vi "Offline_Analysis_SVM_분석기_woF4.vi"(0 "LDA_matrix":path caption="LDA_matrix.txt", 1 "Target":path, 2 "Nontarget":path, 3 "DIscard Channel Info":i32[](array[numeric]), 5 "Target_order.txt":path, 7 "mius_flash_order":path, 9 "Brain":path, 11 "svm_model_file":string, 12 "피험자이름":string="홍길동", 13 "Save_path":string) -> ()   [LabVIEW 2014]
uses:
  <vilib>/Utility/file.llb/Read From Spreadsheet File (DBL).vi
  <vilib>/Analysis/Matrix/Numeric/Conversions/Array To Matrix - RA2.vi
  <vilib>/Analysis/Matrix/Numeric/Conversions/Array To Matrix - RA.vi
  <vilib>/Utility/file.llb/Read From Spreadsheet File (I64).vi
  <vilib>/Utility/file.llb/Write To Spreadsheet File (DBL).vi
  <vilib>/Utility/file.llb/Write To Spreadsheet File (I64).vi
  <vilib>/Utility/file.llb/Write To Spreadsheet File (string).vi
  <vilib>/Analysis/Matrix/NI_Matrix.lvlib
panel:
  out "ACC":i16
  in  "Channel selection":bool[](array[boolean])=[TRUE, TRUE, TRUE, TRUE, TRUE, TRUE, TRUE, TRUE, TRUE, TRUE, TRUE]
  out "Target_order":i64[](array[numeric])
  out "Selected_Target":i32[](array[numeric])
  out "Accuracy":i16[](array[numeric])
  out "error out":errorcluster
  in  "Random_num":i32=6
  in  "Flash_Repeat":i32=20
  in  "Frame_Length":i32=10
  in  "Sampling_Rate":dbl=250.0
  # "ERP_Parameter안씀. LDA바로 집어넣으면 됨"
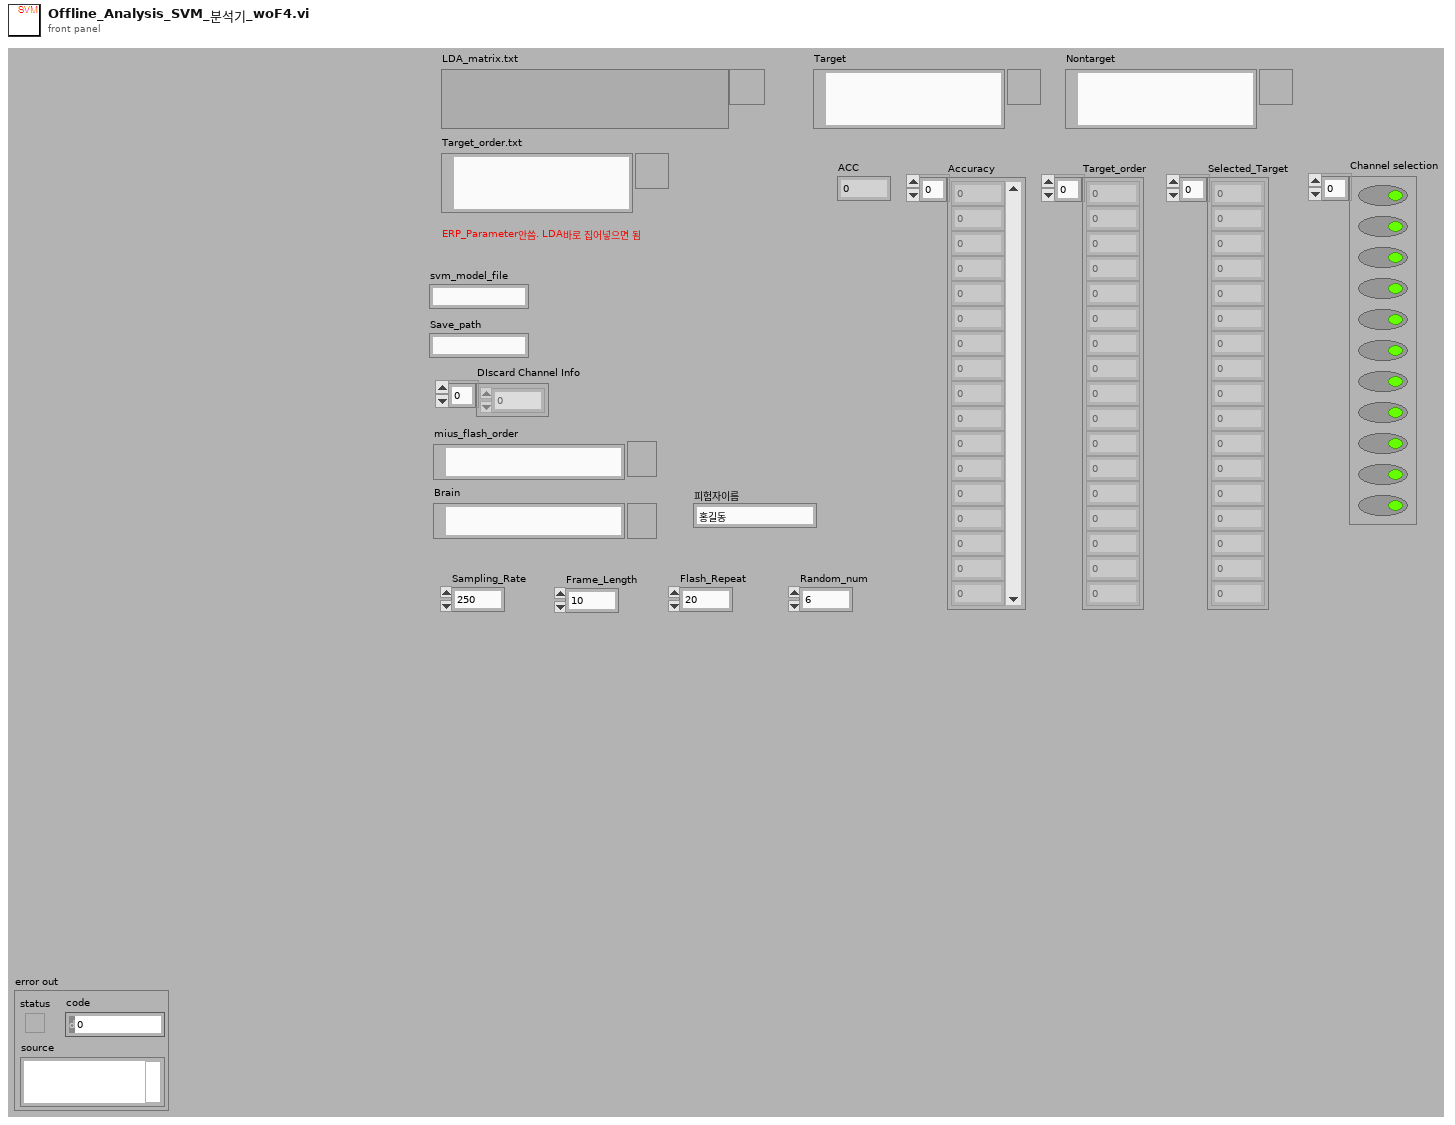
[diagram p1: front panel]
types:
  T1 = typedef "NI_Matrix.lvlib/RealMatrix.ctl" = dbl[][]
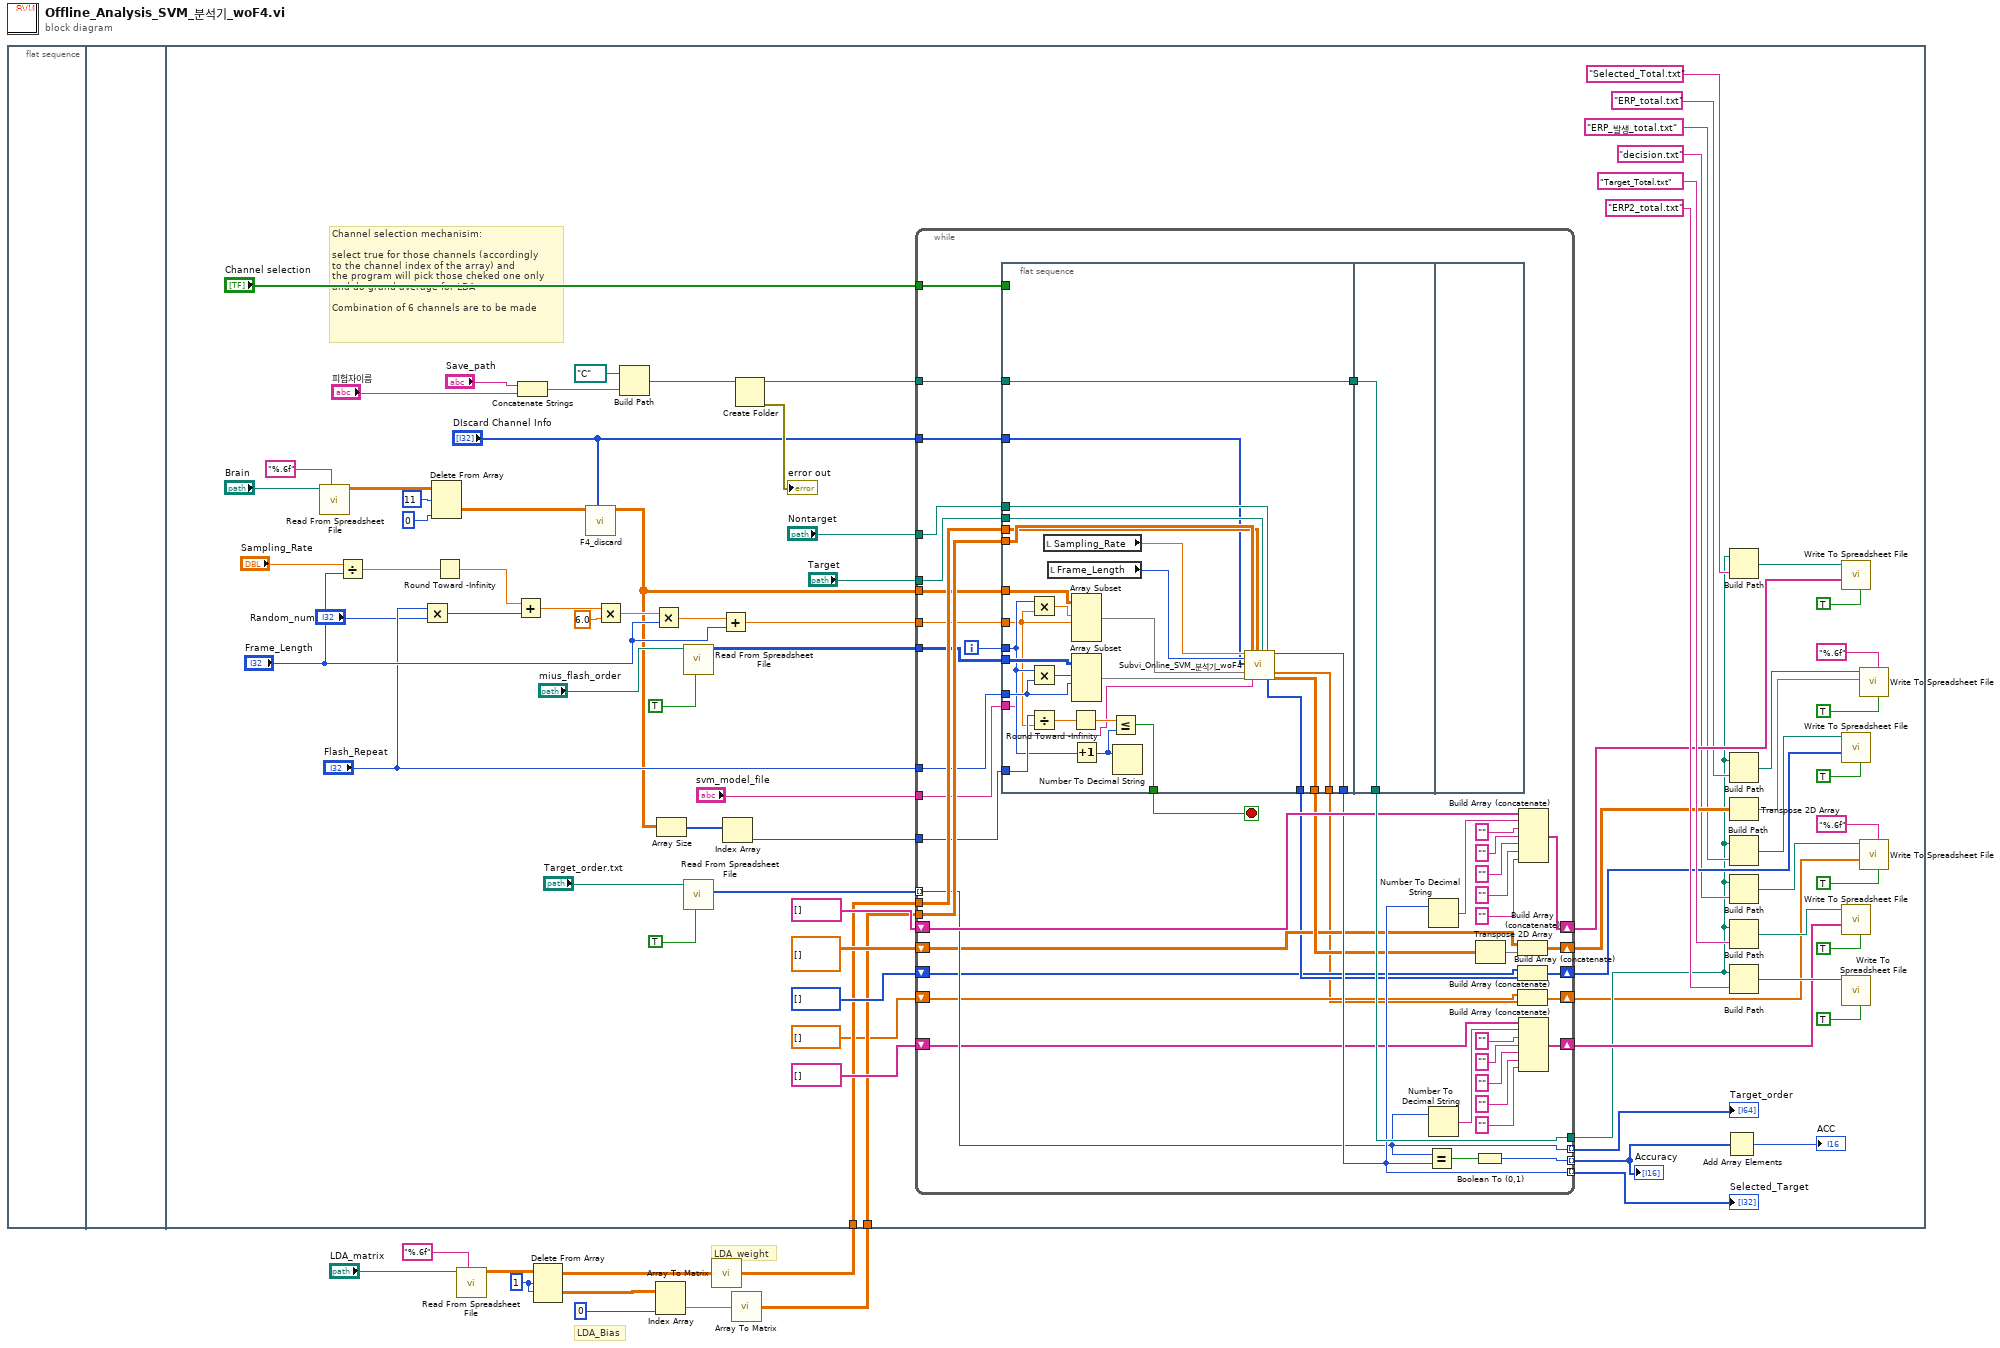
[diagram p0: block diagram]
diagram:
  w5 = 1 ("인덱스 (행)")
  # "LDA_Bias"
  # "LDA_weight"
  n1 = flat-sequence {
    tunnel: w2 -> [w27]
    tunnel: w1 -> [w26]
    frame #0 {
    }
    frame #1 {
    }
    frame #2 {
      # "Channel selection mechanisim:\n\nselect true for those channels (accordingly\nto the channel index of the array) and \nthe program will pick those cheked one only\nand do grand average for LDA\n\nCombination of 6 channels are to be made"
      n2 = call-poly <vilib>:"Read From Spreadsheet File.vi"("format (%.3f)"="%.6f", "file path (dialog if empty)"="Brain") -> ("all rows"=w65:dbl[][])  [unwired: 5 in, 4 out]
      n3 = Divide(x="Sampling_Rate", y="Frame_Length") -> (x/y=w71:dbl)
      n4 = Multiply(x="Flash_Repeat", y="Random_num") -> (x*y=w74:i32)
      n5 = Delete From Array(array=w65, length=11 ("길이"), index (col)=0 ("비활성화된 인덱스 (열)")) -> (deleted portion=w25:dbl[][])  [unwired: 1 in, 1 out]
      n6 = Round Toward -Infinity(1:w71) -> (0:w73:dbl)
      n7 = Add(x=w73, y=w74) -> (x+y=w76:dbl)
      n8 = Concatenate Strings("Save_path", "피험자이름") -> (w17:string)
      n9 = call "F4_discard.vi"("DIscard Channel Info"="DIscard Channel Info", "Array"=w25) -> ("array w/ subset deleted"=w12:dbl[][])  [unwired: 9 in]
      n10 = Multiply(x=w76, y=6.0) -> (x*y=w78:dbl)
      n11 = Build Path(base path=path "C:/" ("path"), name or relative path=w17) -> (appended path=w83:path)
      n12 = Multiply(x=w78, y="Frame_Length") -> (x*y=w80:dbl)
      n13 = Array Size(array=w12) -> (size(s)=w68:i32[])
      n14 = call-poly <vilib>:"Read From Spreadsheet File.vi"("transpose (no:F)"=TRUE, "file path (dialog if empty)"="mius_flash_order") -> ("all rows"=w67:i64[][])  [unwired: 5 in, 4 out]
      n15 = call-poly <vilib>:"Read From Spreadsheet File.vi"("transpose (no:F)"=TRUE, "file path (dialog if empty)"="Target_order.txt") -> ("first row"=w59:i64[])  [unwired: 5 in, 4 out]
      n16 = Add(x=w80, y="Frame_Length") -> (x+y=w81:dbl)
      n17 = Index Array(array=w68) -> (element=w69:i32)  [unwired: 1 in]
      n18 = Create Folder(path (use dialog)=w83) -> (created path=w85:path, error out=→"error out":errorcluster)  [unwired: 2 in, 1 out]
      n19 = while {
        tunnel: w26 -> [w134]
        tunnel: w27 -> [w133]
        tunnel: w12 -> [w131]
        tunnel: w67 -> [w130]
        tunnel: w69 -> [w132]
        tunnel: w81 -> [w128]
        tunnel: "Flash_Repeat" -> [w129]
        tunnel: w85 -> [w127]
        tunnel: w59 -> [w104] mode=indexing
        tunnel: [w124] -> w47 mode=indexing
        tunnel: [w104] -> w56 mode=indexing
        tunnel: [w105] -> w57 mode=indexing
        tunnel: "Channel selection" -> [w121]
        tunnel: [w120] -> w20
        shift-right: [w107] -> w41
        shift-left: string[] [] -> [w106]
        shift-right: [w103] -> w40
        shift-left: string[] [] -> [w102]
        shift-right: [w99] -> w35
        shift-left: dbl[][] [] -> [w98]
        shift-right: [w96] -> w28
        shift-left: i16[] [] -> [w95]
        shift-right: [w94] -> w19
        shift-left: dbl[] [] -> [w93]
        tunnel: "Target" -> [w91]
        tunnel: "Nontarget" -> [w90]
        tunnel: "svm_model_file" -> [w89]
        tunnel: "DIscard Channel Info" -> [w88]
        i -> [w123]
        stop <- w122 stop-if-true
        n20 = flat-sequence {
          tunnel: w134 -> [w161]
          tunnel: w133 -> [w139]
          tunnel: w132 -> [w160]
          tunnel: [w159] -> w122
          tunnel: w131 -> [w158]
          tunnel: w130 -> [w155]
          tunnel: w129 -> [w153]
          tunnel: w123 -> [w152]
          tunnel: w128 -> [w151]
          tunnel: w127 -> [w144]
          tunnel: [w144] -> w126
          tunnel: [w145] -> w105
          tunnel: w121 -> [_]
          tunnel: [w143] -> w101
          tunnel: [w142] -> w97
          tunnel: [w140] -> w92
          tunnel: w91 -> [w138]
          tunnel: w90 -> [w137]
          tunnel: w89 -> [w136]
          tunnel: w88 -> [w135]
          tunnel: w126 -> [w162]
          tunnel: [w162] -> w120
          frame #0 {
            n21 = Multiply(x=w152, y=w151) -> (x*y=w157:dbl)
            n22 = Multiply(x=w152, y=w153) -> (x*y=w154:i32)
            n23 = Divide(x=w160, y=w151) -> (x/y=w150:dbl)
            n24 = local read "Sampling_Rate"() -> (w148:dbl)
            n25 = local read "Frame_Length"() -> (w147:i32)
            n26 = Round Toward -Infinity(1:w150) -> (0:w149:dbl)
            n27 = Array Subset(array=w158, index (row)=w157, length (row)=w151) -> (w156:dbl[][])  [unwired: 2 in]
            n28 = Array Subset(array=w155, index (row)=w154, length (row)=w153) -> (w141:i64[][])  [unwired: 2 in]
            n29 = Increment(x=w152) -> (x+1=w146:i32)
            n30 = Less Or Equal?(x=w149, y=w146) -> (x <= y?=w159:bool)
            n31 = Number To Decimal String(number=w146) -> ()  [unwired: 1 in, 1 out]
            n32 = call "Subvi_Online_SVM_분석기_woF4.vi"("rate"=w148, "samples per channel"=w147, "DIscard Channel Info"=w135, "Brain_data_source"=w156, "Target_Flash_Order"=w141, "Value 2"=w161, "svm_model_file"=w136, "Matrix 2"=w139, "Target"=w138, "Nontarget"=w137) -> ("EPR_발생_total"=w142:i16[], "output-0~8"=w145:i32, "decision"=w140:dbl[], "ERP_Parameters"=w143:dbl[][])  [unwired: 6 in]
          }
          frame #1 {
          }
          frame #2 {
          }
        }
        n33 = Equal?(x=w104, y=w105) -> (x = y?=w125:bool)
        n34 = Number To Decimal String(number=w105) -> (decimal integer string=w113:string)  [unwired: 1 in]
        n35 = Number To Decimal String(number=w104) -> (decimal integer string=w119:string)  [unwired: 1 in]
        n36 = Boolean To (0,1)(Boolean=w125) -> (0, 1=w124:i16)
        n37 = Transpose 2D Array(2D array=w101) -> (transposed array=w100:dbl[][])
        n38 = Build Array (concatenate)(w98, w100) -> (w99:dbl[][])
        n39 = Build Array (concatenate)(w95, w97) -> (w96:i16[])
        n40 = Build Array (concatenate)(w93, w92) -> (w94:dbl[])
        n41 = Build Array (concatenate)(w106, w113, "" ("element"), "" ("element"), "" ("element"), "" ("element"), "" ("element")) -> (w107:string[])
        n42 = Build Array (concatenate)(w102, w119, "" ("element"), "" ("element"), "" ("element"), "" ("element"), "" ("element")) -> (w103:string[])
      }
      "Accuracy" <- w47
      "Selected_Target" <- w57
      "Target_order" <- w56
      n43 = Add Array Elements(numeric array=w47) -> (sum=→"ACC":i16)
      n44 = Build Path(base path=w20, name or relative path="Selected_Total.txt") -> (appended path=w43:path)
      n45 = Build Path(base path=w20, name or relative path="ERP_total.txt") -> (appended path=w36:path)
      n46 = Transpose 2D Array(2D array=w35) -> (transposed array=w33:dbl[][])
      n47 = Build Path(base path=w20, name or relative path="ERP_발생_total.txt") -> (appended path=w30:path)
      n48 = Build Path(base path=w20, name or relative path="decision.txt") -> (appended path=w21:path)
      n49 = Build Path(base path=w20, name or relative path="Target_Total.txt") -> (appended path=w49:path)
      n50 = Build Path(base path=w20, name or relative path="ERP2_total.txt") -> (appended path=w51:path)
      n51 = call-poly <vilib>:"Write To Spreadsheet File.vi"("transpose? (no:F)"=TRUE, "1D data"=w41, "file path (dialog if empty)"=w43) -> ()  [unwired: 5 in, 1 out]
      n52 = call-poly <vilib>:"Write To Spreadsheet File.vi"("transpose? (no:F)"=TRUE, "1D data"=w28, "file path (dialog if empty)"=w30) -> ()  [unwired: 5 in, 1 out]
      n53 = call-poly <vilib>:"Write To Spreadsheet File.vi"("transpose? (no:F)"=TRUE, "1D data"=w40, "file path (dialog if empty)"=w49) -> ()  [unwired: 5 in, 1 out]
      n54 = call-poly <vilib>:"Write To Spreadsheet File.vi"("transpose? (no:F)"=TRUE, "file path (dialog if empty)"=w51) -> ()  [unwired: 6 in, 1 out]
      n55 = call-poly <vilib>:"Write To Spreadsheet File.vi"("transpose? (no:F)"=TRUE, "format (%.3f)"="%.6f", "2D data"=w33, "file path (dialog if empty)"=w36) -> ()  [unwired: 4 in, 1 out]
      n56 = call-poly <vilib>:"Write To Spreadsheet File.vi"("transpose? (no:F)"=TRUE, "format (%.3f)"="%.6f", "1D data"=w19, "file path (dialog if empty)"=w21) -> ()  [unwired: 4 in, 1 out]
    }
  }
  n57 = call-poly <vilib>:"Read From Spreadsheet File.vi"("format (%.3f)"="%.6f", "file path (dialog if empty)"="LDA_matrix") -> ("all rows"=w3:dbl[][])  [unwired: 5 in, 4 out]
  n58 = Delete From Array(array=w3, length=w5, index (row)=w5) -> (deleted portion=w8:dbl[][], array with subset deleted=w7:dbl[][])  [unwired: 1 in]
  n59 = Index Array(array=w8, index (col)=0 ("인덱스")) -> (element=w6:dbl[])  [unwired: 1 in]
  n60 = call-poly <vilib>:"Array To Matrix.vi"("Real 2D Array"=w7) -> ("Real Matrix"=w2:T1)
  n61 = call-poly <vilib>:"Array To Matrix.vi"("Real 1D Array"=w6) -> ("Real Matrix (Column Vector)"=w1:T1)
